vi "GEA2 Send and Receive Message.vi"(0 "GEA2 Reference In":refnum<k24>, 1 "Input Data":T1 {"Command" format="%02x"; "Destination" format="%02x"; "Source" format="%02x"}, 2 "Read Timeout (ms)":u32=500, 5 "Expected Command":string=".*", 7 "Expected Data":string=".*", 9 "Expected Source":string=".*", 11 "Error In":errorcluster, 12 "# of Tries":u8=5 min=1) -> (4 "GEA2 Reference Out":refnum<k24>, 6 "Raw Data Out":string, 8 "Converted Data Out":T2 {"CRC" format="%04x"; "Length" format="%02x"; "Command" format="%02x"; "Destination" format="%02x"; "Source" format="%02x"}, 15 "Error Out":errorcluster)   [LabVIEW 2016, in "GEA2_Toolkit.lvlib"]
doc: "This VI sends and receives data across the GEA2 bus. The VI waits for the expected responses (filtered by the expected command / data fields) or until the timeout occurs."
uses:
  library/GEA2_Toolkit.lvlib
  C:/Users/220038920/Desktop/GEA3 Toolkit/GEA3 DLL Source/GeaCommunication.dll
  GEA3 DLL Source/GeaCommunication.dll
  type defs/Data Out.ctl
  type defs/Data In.ctl
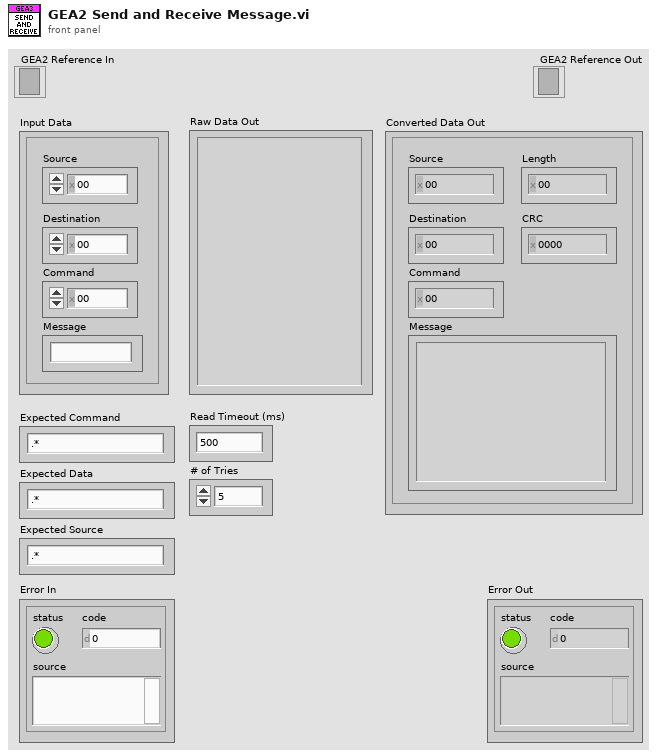
[diagram p1: front panel]
types:
  T1 = typedef "GEA2_Toolkit.lvlib/Data In.ctl" = cluster{"Source":u8, "Destination":u8, "Command":u8, "Message":string}
  T2 = typedef "GEA2_Toolkit.lvlib/Data Out.ctl" = cluster{"Source":u8, "Destination":u8, "Command":u8, "Length":u8, "CRC":u16, "Message":string}
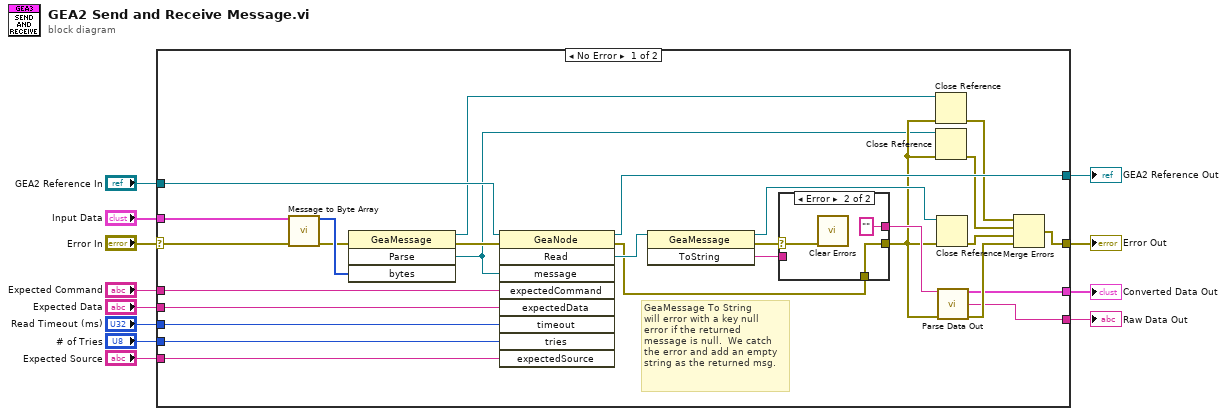
[diagram p0: block diagram]
diagram:
  n1 = case shown="No Error" "Error In" {
    selector: "Error In" -> [w16 w46]
    tunnel: "GEA2 Reference In" -> [w38 w47]
    tunnel: [w30 _] -> w6
    tunnel: [w37 w47] -> w9
    tunnel: [w39 w46] -> w11
    tunnel: "Read Timeout (ms)" -> [w29 _]
    tunnel: [w14 _] -> w7
    tunnel: "Expected Data" -> [w34 _]
    tunnel: "Expected Command" -> [w33 _]
    tunnel: "Input Data" -> [w32 _]
    tunnel: "# of Tries" -> [w24 _]
    tunnel: "Expected Source" -> [w13 _]
    frame No Error {
      # "GeaMessage To String\nwill error with a key null\nerror if the returned\nmessage is null.  We catch\nthe error and add an empty\nstring as the returned msg."
      n2 = call "Message to Byte Array.vi"("Input Data"=w32, "Error In"=w16) -> ("Byte Array"=w21:u8[], "Error Out"=w15:errorcluster)  [unwired: 12 in]
      n3 = invoke class="GeaMessage" method="Parse"(error in=w15, "bytes"=w21) -> (reference out=w20:refnum<k24>, error out=w22:errorcluster, "Parse"=w19:refnum<k24>)  [unwired: 2 in, 1 out]
      n4 = invoke class="GeaNode" method="Read"(reference=w38, error in=w22, "message"=w19, "expectedCommand"=w33, "expectedData"=w34, "timeout"=w29, "tries"=w24, "expectedSource"=w13) -> (reference out=w37:refnum<k24>, error out=w25:errorcluster, "Read"=w28:refnum<k24>)  [unwired: 1 in, 6 out]
      n5 = invoke class="GeaMessage" method="ToString"(reference=w28) -> (reference out=w40:refnum<k24>, error out=w27:errorcluster, "ToString"=w26:string)  [unwired: 2 in]
      n6 = case shown="Error" w27 {
        selector: w27 -> [_ w44]
        tunnel: w26 -> [w42 _]
        tunnel: [w42 "" ("ToString")] -> w31
        tunnel: [w41 w43] -> w23
        tunnel: w25 -> [w41 w43]
        frame No Error {
        }
        frame Error {
          n7 = call <vilib>:"Clear Errors.vi"("error in (no error)"=w44) -> ()  [unwired: 5 in, 2 out]
        }
      }
      n8 = Close Reference(reference=w20, error in (no error)=w23) -> (error out=w17:errorcluster)
      n9 = Close Reference(reference=w19, error in (no error)=w23) -> (error out=w18:errorcluster)
      n10 = Close Reference(reference=w40, error in (no error)=w23) -> (error out=w36:errorcluster)
      n11 = call "Parse Data Out.vi"("Raw Data In"=w31, "Error In"=w23) -> ("Data Out"=w30:T2, "Raw Data Out"=w14:string, "Error Out"=w35:errorcluster)  [unwired: 11 in]
      n12 = Merge Errors(w17, w18, w36, w35) -> (w39:errorcluster)
    }
    frame Error {
    }
  }
  "Raw Data Out" <- w7
  "Error Out" <- w11
  "GEA2 Reference Out" <- w9
  "Converted Data Out" <- w6
